vi "Plot 1 auto meas..vi"(8 "error in (no error)":errorcluster, 9 "App Data":T1, 10 "ref. line [dB]":dbl, 11 "XYGraph in":refnum<vi>) -> (0 "error out":errorcluster)   [LabVIEW 2014]
uses:
  Controls/App Data.ctl
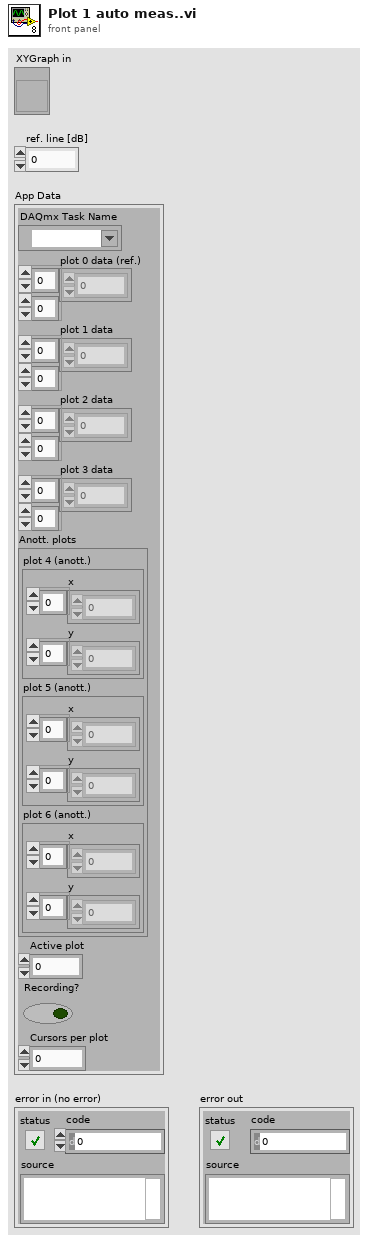
[diagram p1: front panel]
types:
  T1 = typedef "App Data.ctl" = cluster{"DAQmx Task Name":refnum<k21>, "plot 0 data (ref.)":dbl[][], "plot 1 data":dbl[][], "plot 2 data":dbl[][], "plot 3 data":dbl[][], "Anott. plots":cluster{"plot 4 (anott.)":cluster{"x":dbl[], "y":dbl[]}, "plot 5 (anott.)":cluster{"x":dbl[], "y":dbl[]}, "plot 6 (anott.)":cluster{"x":dbl[], "y":dbl[]}}, "Active plot":u32, "Recording?":bool, "Cursors per plot":i32}
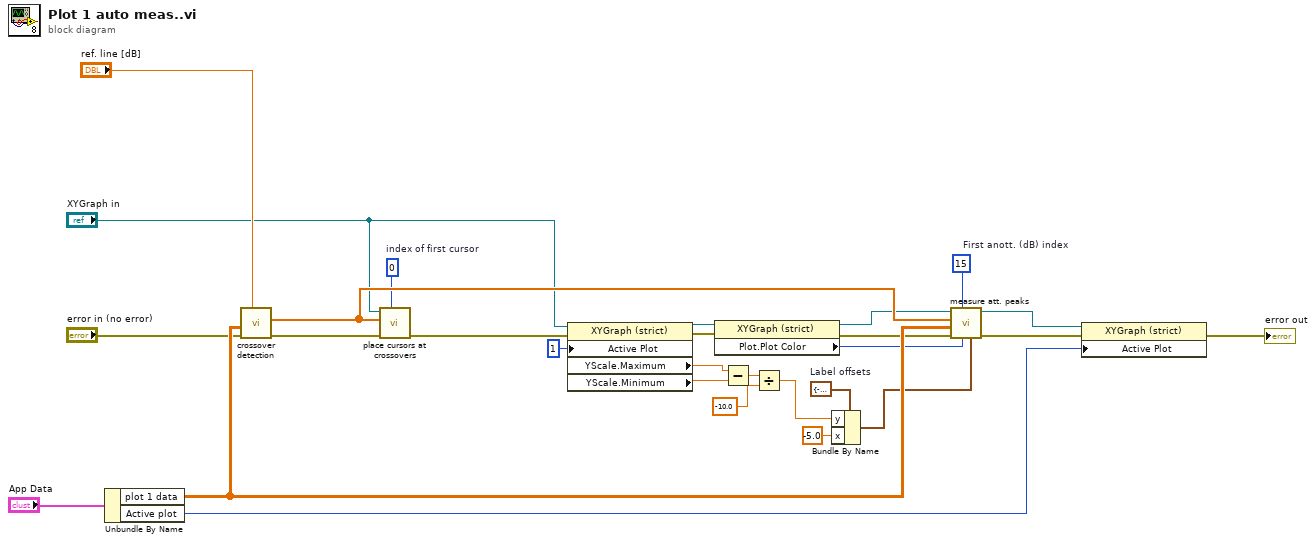
[diagram p0: block diagram]
diagram:
  w2 = cluster{"x":dbl, "y":dbl} {"x"=-5.0, "y"=-0.1}  # Label offsets
  w27 = 15  # First anott. (dB) index
  w23 = 0  # index of first cursor
  n1 = Unbundle By Name("App Data") -> ("plot 1 data"=w26:dbl[][], "Active plot"=w11:u32)
  n2 = call "crossover detection.vi"("reference line"="ref. line [dB]", "error in"="error in (no error)", "Plot"=w26) -> ("error out"=w22:errorcluster, "crossovers"=w25:dbl[])  [unwired: 7 in]
  n3 = call "place cursors at crossovers.vi"("index of first cursor"=w23, "error in (no error)"=w22, "crossovers"=w25, "XYGraph in"="XYGraph in") -> ("error out"=w20:errorcluster)  [unwired: 7 in]
  n4 = property class="XYGraph (strict)"(reference="XYGraph in", error in=w20, "Active Plot"=u32 1) -> (reference out=w17:refnum<vi>, error out=w16:errorcluster, "YScale.Maximum"=w8:dbl, "YScale.Minimum"=w7:dbl)
  n5 = property class="XYGraph (strict)"(reference=w17, error in=w16) -> (reference out=w15:refnum<vi>, error out=w14:errorcluster, "Plot.Plot Color"=w10:u32)
  n6 = Subtract(x=w8, y=w7) -> (x-y=w6:dbl)
  n7 = Divide(x=w6, y=-10.0) -> (x/y=w4:dbl)
  n8 = Bundle By Name(cluster=w2, "y"=w4, "x"=-5.0) -> (w1:cluster{"x":dbl, "y":dbl})
  n9 = call "measure att. peaks.vi"("Label offsets"=w1, "Peak annot. color"=w10, "First anott. index"=w27, "error in"=w14, "Plot"=w26, "crossovers"=w25, "XYGraph in"=w15) -> ("error out"=w12:errorcluster, "XYGraph out"=w13:refnum<vi>)  [unwired: 3 in]
  n10 = property class="XYGraph (strict)"(reference=w13, error in=w12, "Active Plot"=w11) -> (error out=→"error out":errorcluster)  [unwired: 1 out]
